vi "Generate TimeSeries folder.vi"(8 "error in (no error)":errorcluster) -> (0 "error out":errorcluster, 3 "Timelapse folder path":path)   [LabVIEW 2020]
uses:
  Typedefs/Experiment folder base name.ctl
  Global Variables/General Globals.vi
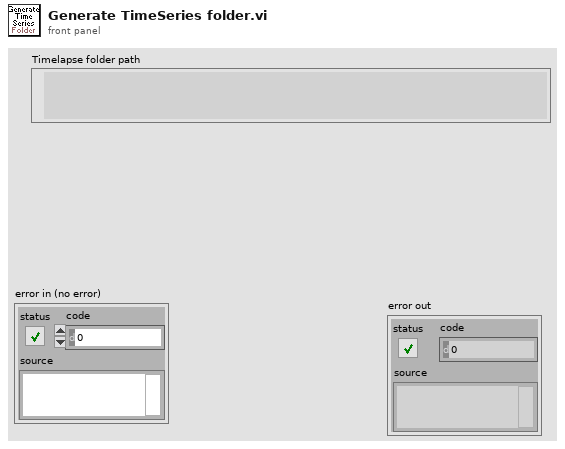
[diagram p1: front panel]
types:
  T1 = typedef "Experiment folder base name.ctl" = enum16{"TimeLapse", "FunctAcq"}
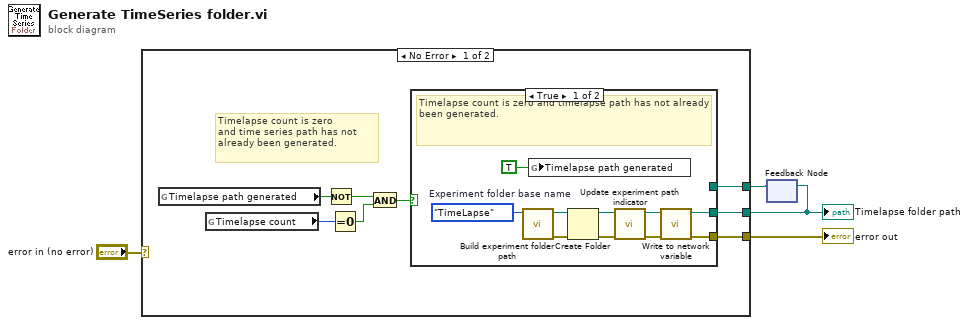
[diagram p0: block diagram]
diagram:
  n1 = feedback #1() -> (w1:path)  [unwired: 1 in]
  n2 = case shown="No Error" "error in (no error)" {
    selector: "error in (no error)" -> [_ w24]
    tunnel: [w12 w24] -> w4
    tunnel: [w11 w25] -> w2
    tunnel: w1 -> [w9 w25]
    frame No Error {
      # "Timelapse count is zero\nand time series path has not already been generated."
      n3 = global read "General Globals.vi" "Timelapse path generated"() -> (w7:bool)
      n4 = global read "General Globals.vi" "Timelapse count"() -> (w8:u32)
      n5 = Not(x=w7) -> (.not. x?=w6:bool)
      n6 = Equal To 0?(x=w8) -> (x = 0?=w5:bool)
      n7 = And(x=w6, y=w5) -> (x .and. y?=w10:bool)
      n8 = case shown="True" w10 {
        tunnel: [w20 w23] -> w11
        tunnel: [w21 _] -> w12
        tunnel: w9 -> [_ w23]
        frame True {
          w13 = Experiment_folder_base_name."TimeLapse"  # Experiment folder base name
          # "Timelapse count is zero and timelapse path has not already been generated."
          n9 = call "Build experiment folder path.vi"("Experiment folder base name"=w13) -> ("error out"=w15:errorcluster, "Experiment folder  file path"=w17:path)  [unwired: 9 in]
          n10 = global write "General Globals.vi" "Timelapse path generated"(TRUE ("Timelapse path generated")) -> ()
          n11 = Create Folder(path (use dialog)=w17, error in=w15) -> (created path=w16:path, error out=w14:errorcluster)  [unwired: 1 in, 1 out]
          n12 = call "Update experiment path indicator.vi"("error in (no error)"=w14, "created path"=w16) -> ("error out"=w18:errorcluster, "created path (dup)"=w19:path)  [unwired: 8 in]
          n13 = call "Write to network variable.vi"("error in (no error)"=w18, "created path"=w19) -> ("error out"=w21:errorcluster, "created path (dup)"=w20:path)  [unwired: 8 in]
        }
        frame False {
        }
      }
    }
    frame Error {
    }
  }
  "Timelapse folder path" <- w2
  "error out" <- w4
  n14 = feedback-in #1(w2) -> ()
